vi "ziGetVoltageParams.vi"(1 "Extra Gain":dbl=1.0, 7 "ZCtrl (0)":dbl, 8 "Error In":errorcluster, 9 "Demodulator (0)":i32, 10 "Mode":enum16{"From Sig Out", "Signal Input", "HF2CA"}(ring), 11 "Handle In":T1 {"Handle" format="0x%08x"; "Conn" format="0x%08x"}) -> (0 "Error Out":errorcluster, 2 "VGain":dbl, 3 "Handle Out":T1 {"Handle" format="0x%08x"; "Conn" format="0x%08x"}, 4 "Vz (Vrms)":cdb format="%#_6p", 6 "Imp50":bool)   [LabVIEW 2015, in "Zurich Instruments LabOne.lvlib"]
uses:
  Zurich Instruments LabOne.lvlib
  ziTypeHandle.ctl
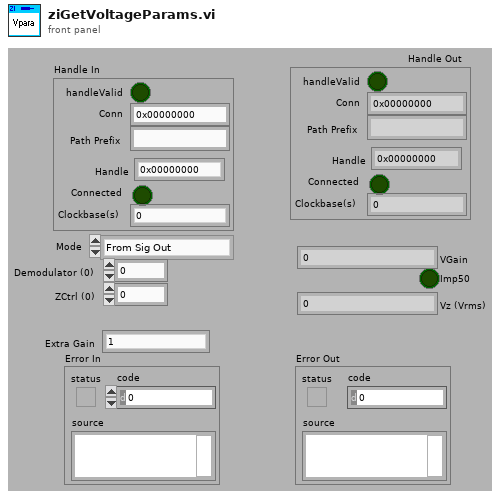
[diagram p1: front panel]
types:
  T1 = typedef "Zurich Instruments LabOne.lvlib/ziTypeHandle.ctl" = cluster{"handleValid":bool, "Conn":u64, "Path Prefix":string, "Handle":u64, "Connected":bool, "Clockbase(s)":dbl}
  T2 = cluster{"Timestamps (ticks)":u64, "X (Vrms)":dbl, "Y (Vrms)":dbl, "Osc Phase (deg)":dbl, "Freq (Hz)":dbl, "DIO":u32, "AuxIn0 (V)":dbl, "AuxIn1 (V)":dbl}
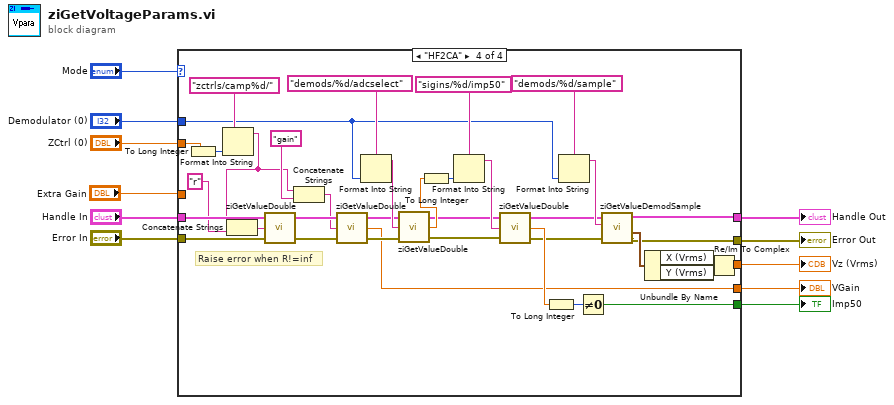
[diagram p0: block diagram]
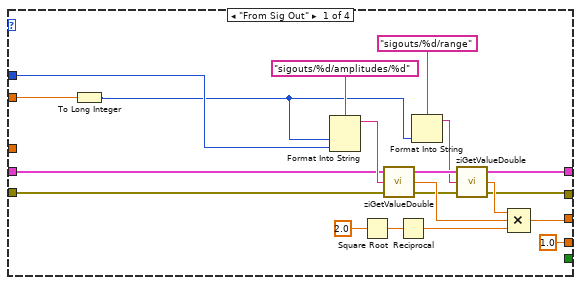
[diagram p2: hidden frame]
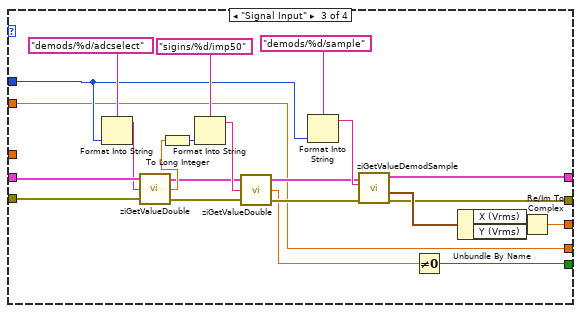
[diagram p4: hidden frame]
diagram:
  n1 = case shown="\"HF2CA\"" "Mode" {
    tunnel: "ZCtrl (0)" -> [w13 _ w34 w65]
    tunnel: "Handle In" -> [w16 w33 w41 w94]
    tunnel: [w27 w33 w52 w89] -> w4
    tunnel: "Demodulator (0)" -> [w17 _ w38 w76]
    tunnel: "Error In" -> [w15 w32 w42 w83]
    tunnel: [w26 w32 w51 w82] -> w6
    tunnel: [w29 _ w50 w74] -> w11
    tunnel: [_ _ w36 w59] -> w9
    tunnel: [1.0 ("Value") _ w34 w66] -> w10
    tunnel: "Extra Gain" -> [_ _ _ _]
    frame "From Sig Out" {
      n2 = To Long Integer(number=w13) -> (32bit integer=w12:i32)
      n3 = Format Into String(format string="sigouts/%d/amplitudes/%d", w12, w17) -> (resulting string=w21:string)  [unwired: 2 in, 1 out]
      n4 = Square Root(x=2.0) -> (sqrt(x)=w20:dbl)
      n5 = call "ziGetValueDouble.vi"("error in"=w15, "Path"=w21, "Handle in"=w16) -> ("error out"=w23:errorcluster, "Value"=w25:dbl, "Handle out"=w24:T1)
      n6 = Reciprocal(x=w20) -> (1/x=w18:dbl)
      n7 = Format Into String(format string="sigouts/%d/range", w12) -> (resulting string=w22:string)  [unwired: 2 in, 1 out]
      n8 = call "ziGetValueDouble.vi"("error in"=w23, "Path"=w22, "Handle in"=w24) -> ("error out"=w26:errorcluster, "Value"=w28:dbl, "Handle out"=w27:T1)
      n9 = Compound Arithmetic op=MULTIPLY(w28, w25, w18) -> (w29:dbl)
    }
    frame Default {
    }
    frame "Signal Input" {
      n10 = Format Into String(format string="demods/%d/adcselect", w38) -> (resulting string=w37:string)  [unwired: 2 in, 1 out]
      n11 = call "ziGetValueDouble.vi"("error in"=w42, "Path"=w37, "Handle in"=w41) -> ("error out"=w45:errorcluster, "Value"=w46:dbl, "Handle out"=w44:T1)
      n12 = To Long Integer(number=w46) -> (32bit integer=w43:i32)
      n13 = Format Into String(format string="sigins/%d/imp50", w43) -> (resulting string=w48:string)  [unwired: 2 in, 1 out]
      n14 = call "ziGetValueDouble.vi"("error in"=w45, "Path"=w48, "Handle in"=w44) -> ("error out"=w39:errorcluster, "Value"=w35:dbl, "Handle out"=w40:T1)
      n15 = Format Into String(format string="demods/%d/sample", w38) -> (resulting string=w53:string)  [unwired: 2 in, 1 out]
      n16 = call "ziGetValueDemodSample.vi"("error in"=w39, "Path"=w53, "Handle In"=w40) -> ("error out"=w51:errorcluster, "Demod Sample Out"=w57:T2, "Handle Out"=w52:T1)  [unwired: 2 in]
      n17 = Not Equal To 0?(x=w35) -> (x != 0?=w36:bool)
      n18 = Unbundle By Name(w57) -> ("X (Vrms)"=w55:dbl, "Y (Vrms)"=w56:dbl)
      n19 = Re/Im To Complex(1:w56, 2:w55) -> (0:w50:cdb)
    }
    frame "HF2CA" {
      # "Raise error when R!=inf"
      n20 = To Long Integer(number=w65) -> (32bit integer=w58:i32)
      n21 = Format Into String(format string="zctrls/camp%d/", w58) -> (resulting string=w62:string)  [unwired: 2 in, 1 out]
      n22 = Concatenate Strings(w62, "r") -> (w60:string)
      n23 = call "ziGetValueDouble.vi"("error in"=w83, "Path"=w60, "Handle in"=w94) -> ("error out"=w69:errorcluster, "Handle out"=w70:T1)  [unwired: 1 out]
      n24 = Concatenate Strings(w62, "gain") -> (w61:string)
      n25 = call "ziGetValueDouble.vi"("error in"=w69, "Path"=w61, "Handle in"=w70) -> ("error out"=w68:errorcluster, "Value"=w66:dbl, "Handle out"=w67:T1)
      n26 = Format Into String(format string="demods/%d/adcselect", w76) -> (resulting string=w75:string)  [unwired: 2 in, 1 out]
      n27 = call "ziGetValueDouble.vi"("error in"=w68, "Path"=w75, "Handle in"=w67) -> ("error out"=w79:errorcluster, "Value"=w80:dbl, "Handle out"=w78:T1)
      n28 = To Long Integer(number=w80) -> (32bit integer=w77:i32)
      n29 = Format Into String(format string="sigins/%d/imp50", w77) -> (resulting string=w91:string)  [unwired: 2 in, 1 out]
      n30 = call "ziGetValueDouble.vi"("error in"=w79, "Path"=w91, "Handle in"=w78) -> ("error out"=w71:errorcluster, "Value"=w90:dbl, "Handle out"=w72:T1)
      n31 = To Long Integer(number=w90) -> (32bit integer=w73:i32)
      n32 = Format Into String(format string="demods/%d/sample", w76) -> (resulting string=w84:string)  [unwired: 2 in, 1 out]
      n33 = Not Equal To 0?(x=w73) -> (x != 0?=w59:bool)
      n34 = call "ziGetValueDemodSample.vi"("error in"=w71, "Path"=w84, "Handle In"=w72) -> ("error out"=w82:errorcluster, "Demod Sample Out"=w88:T2, "Handle Out"=w89:T1)  [unwired: 2 in]
      n35 = Unbundle By Name(w88) -> ("X (Vrms)"=w86:dbl, "Y (Vrms)"=w87:dbl)
      n36 = Re/Im To Complex(1:w87, 2:w86) -> (0:w74:cdb)
    }
  }
  "Vz (Vrms)" <- w11
  "VGain" <- w10
  "Imp50" <- w9
  "Error Out" <- w6
  "Handle Out" <- w4
